vi "Analyzer_Proto.vi"() -> ()   [LabVIEW 2012]
uses:
  <vilib>/addons/Wavelet Analysis/typedefs.llb/WA Data.ctl
  <vilib>/addons/Time Frequency Analysis/typedefs.llb/TFA Data.ctl
  <vilib>/addons/Wavelet Analysis/filter banks.llb/WA 1D Analysis Filter Bank (Waveform).vi
  <vilib>/addons/_Advanced Signal Processing/NI_AdvSigProcWA.lvlib
  <vilib>/addons/_Advanced Signal Processing/NI_AdvSigProcTFA.lvlib
  <vilib>/addons/Wavelet Analysis/discrete wavelet transform.llb/WA 1D Discrete Wavelet Transform (Waveform).vi
  <vilib>/addons/Wavelet Analysis/discrete wavelet transform.llb/WA Inverse 1D Discrete Wavelet Transform (Waveform).vi
panel:
  out "Array":string[](array[string])
  in  "level":i32=1
  out "Numeric":i32
  out "Waveform Graph":waveform(dbl)[](graph)
  in  "Select":bool
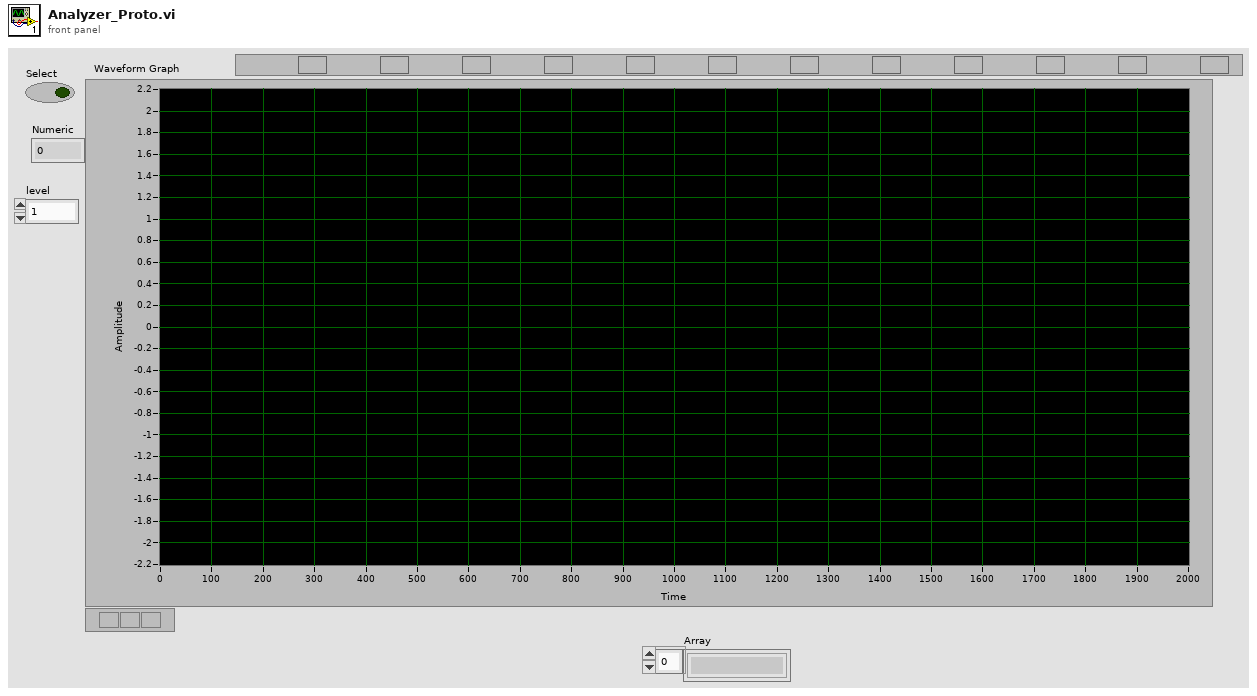
[diagram p1: front panel]
types:
  T1 = typedef "NI_AdvSigProcTFA.lvlib/TFA Data.ctl" = u16
  T2 = typedef "NI_AdvSigProcWA.lvlib/WA Data.ctl" = u16
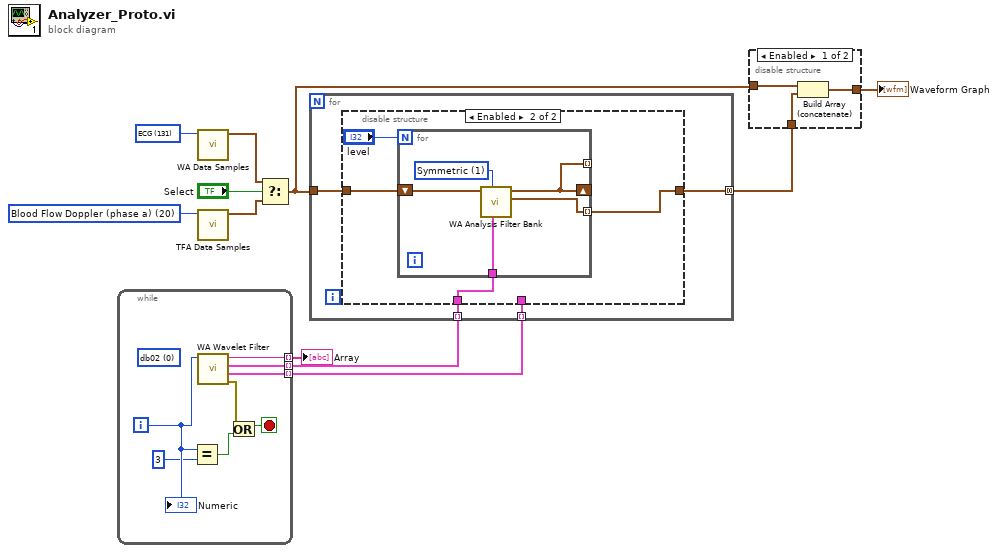
[diagram p0: block diagram]
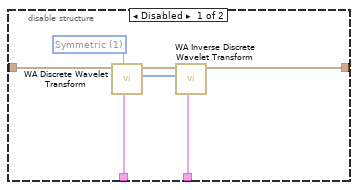
[diagram p3: hidden frame]
diagram:
  w10 = T1 20 items=["PC Fan"=0, "Noisy Chirps"=1, "TDR 1"=2, "TDR 2"=3, "Liquefaction"=4, "Liquefaction Free"=5, "Aneurysm"=6, "Bat"=7, "RF"=8, "Two Gaussian"=9, "Three Gaussian"=10, "Chirp"=11, "Gaussian Chirp"=12, "Cross Chirp"=13, "Doppler"=14, "HOP"=15, "TF Sine"=16, "Three Tone"=17, "Four Tone"=23, "Blood Flow Doppler (phase a)"=20, "Blood Flow Doppler (phase b)"=21, "Heart sound"=22, "-"=18, "Random Noise"=19] ("data")
  w11 = T2 131 items=["1D Example Data"=100, "-"=101, "Doppler"=102, "HOP"=103, "TF Sine"=104, "Noisy Doppler"=105, "Sea Temperature"=106, "Sp500"=107, "Power Line"=108, "Engine Knocking"=109, "HeaviSine"=110, "Bumps"=111, "Blocks"=112, "Piece Regular"=113, "HypChirps"=114, "LinChirps"=115, "Chirps"=116, "Piece Polynomial"=117, "ECG"=131, "-"=118, "2D Example Data"=119, "-"=120, "Finger Print (Image)"=121, "Iris Flower (Image)"=122, "Mammogram (Image)"=123, "Lake (Image)"=127, "Two Can 1 (Image)"=132, "Two Can 2 (Image)"=133, "Camera Man (Image)"=134] ("data")
  n1 = while {
    tunnel: [w18] -> w4 mode=indexing
    tunnel: [w17] -> w3 mode=indexing
    tunnel: [w16] -> w1 mode=indexing
    i -> [w15]
    stop <- w13 stop-if-true
    (unwired) u16 0 items=["db02"=0, "db03"=1, "db04"=2, "db05"=3, "db06"=4, "db07"=5, "db08"=6, "db09"=7, "db10"=8, "db11"=9, "db12"=10, "db13"=11, "db14"=12, "Haar"=13, "bior1_3"=14, "bior1_5"=15, "bior2_2"=16, "bior2_4"=17, "bior2_6"=18, "bior2_8"=19, "bior3_1"=20, "bior3_3"=21, "bior3_5"=22, "bior3_7"=23, "bior3_9"=24, "bior4_4 (FBI)"=25, "bior5_5"=38, "bior6_8"=39, "coif1"=26, "coif2"=27, "coif3"=28, "coif4"=29, "coif5"=30, "sym2"=31, "sym3"=32, "sym4"=33, "sym5"=34, "sym6"=35, "sym7"=36, "sym8"=37] ("wavelet")
    n2 = Equal?(x=w15, y=3) -> (x = y?=w12:bool)
    n3 = call <vilib>:"WA Wavelet Filter.vi"("wavelet"=w15) -> ("error out"=w19:errorcluster, "synthesis filters"=w17:cluster{"lowpass":dbl[], "highpass":dbl[]}, "analysis filters"=w18:cluster{"lowpass":dbl[], "highpass":dbl[]}, "wavelet name"=w16:string)  [unwired: 7 in]
    n4 = Or(x=w19, y=w12) -> (x .or. y?=w13:bool)
    "Numeric" <- w15
  }
  "Array" <- w1
  n5 = call <vilib>:"WA Data Samples.vi"("data"=w11) -> ("signal"=w9:waveform(dbl))  [unwired: 9 in, 1 out]
  n6 = call <vilib>:"TFA Data Samples.vi"("data"=w10) -> ("signal"=w8:waveform(dbl))  [unwired: 9 in, 1 out]
  n7 = Select(t=w9, s="Select", f=w8) -> (s? t:f=w5:waveform(dbl))
  n8 = for {
    tunnel: w5 -> [w23]
    tunnel: w4 -> [w22] mode=indexing
    tunnel: w3 -> [w21] mode=indexing
    tunnel: [w20] -> w2 mode=concatenating
    n9 = disable-structure shown="Enabled" {
      disable-tunnel: w23 -> [w30 w34]
      disable-tunnel: w22 -> [w28 w33]
      disable-tunnel: w21 -> [w25 _]
      disable-tunnel: [w24 w32] -> w20
      frame Disabled {
        w29 = u16 1 items=["Zero padding", "Symmetric", "Periodic"] ("extension")
        n10 = call-poly <vilib>:"WA Discrete Wavelet Transform.vi"("analysis filters"=w28, "extension"=w29, "signal"=w30) -> ("length"=w26:i32[], "DWT coef"=w27:waveform(dbl))  [unwired: 6 in, 1 out]
        n11 = call-poly <vilib>:"WA Inverse Discrete Wavelet Transform.vi"("synthesis filters"=w25, "length"=w26, "DWT coef"=w27) -> ("signal"=w24:waveform(dbl))  [unwired: 7 in, 1 out]
      }
      frame Enabled {
        n12 = for {
          N: "level" -> [_]
          tunnel: w33 -> [w38]
          tunnel: [w36] -> w32 mode=indexing
          shift-right: [w35] -> _
          shift-left: w34 -> [w39]
          tunnel: [w35] -> _ mode=indexing
          w37 = u16 1 items=["Zero padding", "Symmetric", "Periodic"] ("extension")
          n13 = call-poly <vilib>:"WA Analysis Filter Bank.vi"("analysis filters"=w38, "extension"=w37, "signal"=w39) -> ("detail coef"=w36:waveform(dbl), "approx coef"=w35:waveform(dbl))  [unwired: 6 in, 1 out]
        }
      }
    }
  }
  n14 = disable-structure shown="Enabled" {
    disable-tunnel: [w42 w43] -> w6
    disable-tunnel: w5 -> [w41 _]
    disable-tunnel: w2 -> [w40 w43]
    frame Enabled {
      n15 = Build Array (concatenate)(w41, w40) -> (w42:waveform(dbl)[])
    }
    frame Disabled {
    }
  }
  "Waveform Graph" <- w6
